vi "Asylum_Driver_LithographyObjectDots.vi"(4 "Abort Notifier":refnum<notifier>, 6 "Interpolation":dbl format="%#_13g", 7 "Writing Setpoint":dbl=0.1 format="%#_13g", 8 "error in (no error)":errorcluster, 9 "Offsets":cluster{"X":dbl, "Y":dbl}, 10 "Pattern Data":T2={"Name"="", "Litho"=[], "Set Resistance"=enum."1G ohm", "Meta"=variant}, 11 "Application":refnum<k7>) -> (0 "error out":errorcluster, 1 "Y":dbl[](array[numeric]), 2 "X":dbl[](array[numeric]), 3 "Application":refnum<k7>)   [LabVIEW 2019]
uses:
  <userlib>/LevyLab/Relay Box/Typedefs/Resistor--enum.ctl
  <userlib>/LevyLab/Relay Box/Relay-Box.lvclass
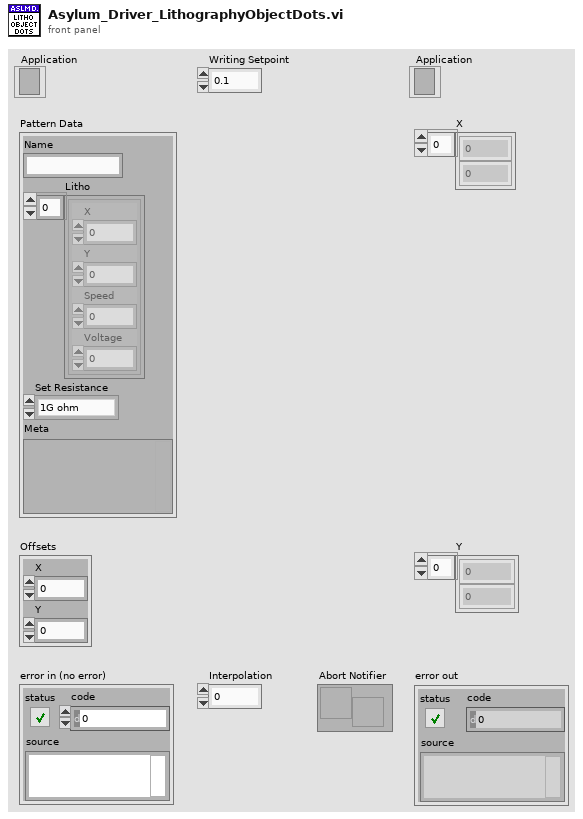
[diagram p1: front panel]
types:
  T1 = typedef "Relay-Box.lvclass/Resistor--enum.ctl" = enum16{"open", "discharge tip", "0 ohms", "100k ohm", "10M ohm", "1G ohm"}
  T2 = cluster{"Name":string, "Litho":cluster{"X":dbl, "Y":dbl, "Speed":dbl, "Voltage":dbl}[], "Set Resistance":T1, "Meta":variant}
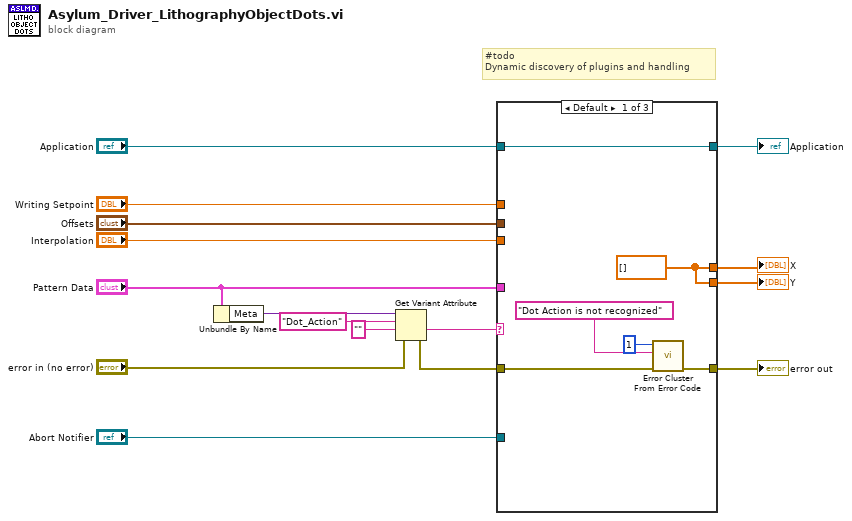
[diagram p0: block diagram]
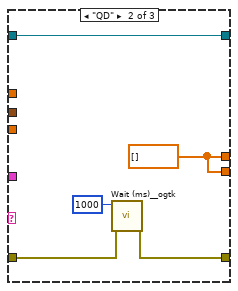
[diagram p2: hidden frame]
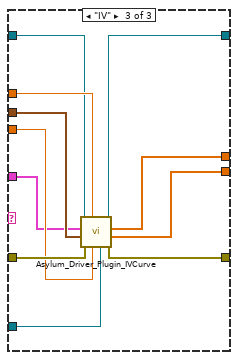
[diagram p3: hidden frame]
diagram:
  # "#todo\nDynamic discovery of plugins and handling"
  n1 = Unbundle By Name("Pattern Data") -> ("Meta"=w14:variant)
  n2 = Get Variant Attribute(Variant=w14, name="Dot_Action", default value (empty Variant)="", error in="error in (no error)") -> (value=w12:string, error out=w7:errorcluster)  [unwired: 2 out]
  n3 = case shown="Default" w12 {
    tunnel: [w22 w25 w37] -> w16
    tunnel: w7 -> [w19 w24 w38]
    tunnel: "Application" -> [w20 w27 w31]
    tunnel: [w20 w27 w32] -> w10
    tunnel: "Pattern Data" -> [_ _ w33]
    tunnel: "Abort Notifier" -> [_ _ w30]
    tunnel: "Writing Setpoint" -> [_ _ w34]
    tunnel: "Offsets" -> [_ _ w35]
    tunnel: "Interpolation" -> [_ _ w36]
    tunnel: [w18 w26 w29] -> w2
    tunnel: [w18 w26 w28] -> w1
    frame Default {
      w18 = dbl[] [] ("X")
      n4 = call <vilib>:"Error Cluster From Error Code.vi"("error in (no error)"=w19, "error message (\"\")"="Dot Action is not recognized" ("error message (\"\")"), "error code (0)"=1) -> ("error out"=w22:errorcluster)  [unwired: 6 in]
    }
    frame "QD" {
      w26 = dbl[] [] ("X")
      n5 = call <userlib>:"Wait (ms)__ogtk.vi"("error in (no error)"=w24, "milliseconds to wait"=u32 1000) -> ("error out"=w25:errorcluster)  [unwired: 8 in, 1 out]
    }
    frame "IV" {
      n6 = call "Asylum_Driver_Plugin_IVCurve.vi"("Abort Notifier"=w30, "Interpolation"=w36, "Writing Setpoint"=w34, "error in (no error)"=w38, "Offsets"=w35, "Pattern Data"=w33, "Application"=w31) -> ("error out"=w37:errorcluster, "Y"=w28:dbl[], "X"=w29:dbl[], "Application Out"=w32:refnum<k7>)  [unwired: 1 in]
    }
  }
  "error out" <- w16
  "Application" <- w10
  "Y" <- w1
  "X" <- w2
